vi "Publish Panel Resized.vi"(8 "error in (no error)":errorcluster, 10 "Rectangle":T1, 11 "Flex  Dialog (Actor) in":refnum<class "Flex Dialog (Actor).lvclass">) -> (0 "error out":errorcluster, 3 "Flex  Dialog (Actor) out":refnum<class "Flex Dialog (Actor).lvclass">)   [LabVIEW 2016, in "Flex UI Dialog (Actor).lvlib" / "Flex Dialog (Actor).lvclass"]
uses:
  Flex Dialog (Actor).lvclass
  <vilib>/East West Architects/MVC Subscription/Subscription/MVC Subscription.lvclass
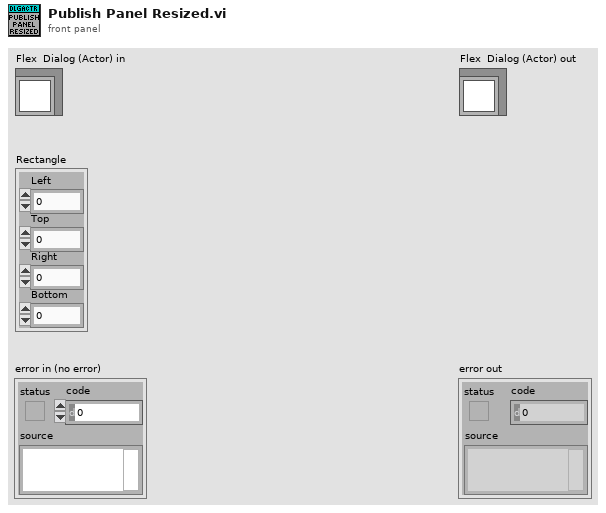
[diagram p1: front panel]
types:
  T1 = cluster{"Left":i16, "Top":i16, "Right":i16, "Bottom":i16}
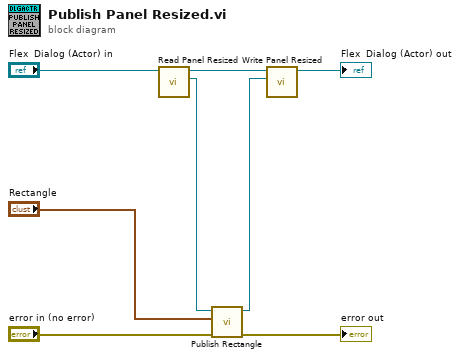
[diagram p0: block diagram]
diagram:
  n1 = call-dynamic "Read Panel Resized.vi"("Flex  Dialog (Actor) in"="Flex  Dialog (Actor) in") -> ("Panel Resized"=w4:refnum<class "MVC Subscription.lvclass">, "Flex  Dialog (Actor) out"=w6:refnum<class "Flex Dialog (Actor).lvclass">)  [unwired: 9 in]
  n2 = call <vilib>:"Publish Rectangle.vi"("error in (no error)"="error in (no error)", "Rectangle"="Rectangle", "MVC Subscription in"=w4) -> ("error out"=→"error out":errorcluster, "MVC Subscription out"=w1:refnum<class "MVC Subscription.lvclass">)  [unwired: 7 in]
  n3 = call-dynamic "Write Panel Resized.vi"("Panel Resized"=w1, "Flex  Dialog (Actor) in"=w6) -> ("Flex  Dialog (Actor) out"=→"Flex  Dialog (Actor) out":refnum<class "Flex Dialog (Actor).lvclass">)  [unwired: 9 in]
